vi "Velocity  실습.vi"() -> ()   [LabVIEW 2014]
uses:
  <vilib>/Motion/FlexMotion/CustomControls/CustomControls.llb/AxisOrVectorSpace To Configure.flx
  <vilib>/Motion/FlexMotion/FunctionsVIs/Trajectory.llb/Load Acceleration/Deceleration.flx
  <vilib>/Motion/FlexMotion/FunctionsVIs/StartStopMotion.llb/Start Motion (8 axes).flx
  <vilib>/Motion/FlexMotion/FunctionsVIs/StartStopMotion.llb/Stop Motion (8 axes).flx
panel:
  in  "정지":bool
  in  "Velocity (10000)":i32=3600 min=-20000000 max=20000000
  in  "Acceleration (100000)":u32=36000
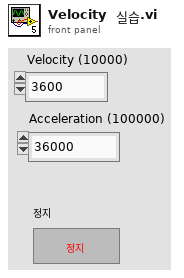
[diagram p1: front panel]
types:
  T1 = enum16{"Absolute Position", "Relative Position", "Velocity", "Relative to Cap Pos", "Modulus Position", "Absolute Contouring", "Relative Contouring"}
  T2 = typedef "AxisOrVectorSpace To Configure.flx" = u16
  T3 = typedef "Resource Out (Enum).flx" = u16
  T4 = typedef "Bd Id Out" = u8
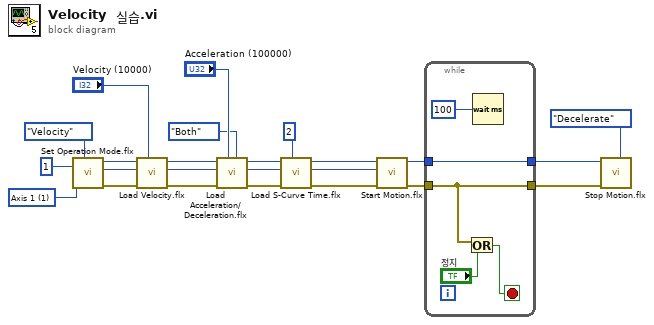
[diagram p0: block diagram]
diagram:
  w24 = T2 1 items=["Axis 1"=1, "Axis 2"=2, "Axis 3"=3, "Axis 4"=4, "Axis 5"=5, "Axis 6"=6, "Axis 7"=7, "Axis 8"=8, "Vector Space 1"=17, "Vector Space 2"=18, "Vector Space 3"=19, "Vector Space 4"=20] ("Axis or Vector Space")
  n1 = call <vilib>:"Set Operation Mode.flx"("Position Mode (Absolute)"=T1."Velocity", "Axis or Vector Space"=w24, "Board ID"=u8 1) -> ("error out"=w12:errorcluster, "Resource Output"=w13:T3, "Bd ID Out"=w14:T4)  [unwired: 3 in]
  n2 = call <vilib>:"Load Velocity.flx"("Velocity (10000)"="Velocity (10000)", "error in (no error)"=w12, "Axis or Vector Space"=w13, "Board ID"=w14) -> ("error out"=w8:errorcluster, "Resource Output"=w9:T3, "Bd ID Out"=w10:T4)  [unwired: 3 in]
  n3 = call "Load Acceleration/Deceleration.flx"("Acceleration Type (Both)"=enum16{"Both", "Acceleration", "Deceleration"}."Both", "Acceleration (100000)"="Acceleration (100000)", "error in (no error)"=w8, "Axis or Vector Space"=w9, "Board ID"=w10) -> ("error out"=w18:errorcluster, "Resource Output"=w19:T3, "Bd ID Out"=w20:T4)  [unwired: 2 in]
  n4 = call <vilib>:"Load S-Curve Time.flx"("S Curve Time (1)"=u16 2, "error in (no error)"=w18, "Axis or Vector Space"=w19, "Board ID"=w20) -> ("error out"=w5:errorcluster, "Resource Output"=w6:T3, "Bd ID Out"=w17:T4)  [unwired: 3 in]
  n5 = call-poly <vilib>:"Start Motion.flx"("error in (no error)"=w5, "Axis or Vector Space"=w6, "Board ID"=w17) -> ("error out"=w2:errorcluster, "Bd ID Out"=w16:T4)  [unwired: 3 in, 1 out]
  n6 = while {
    tunnel: w16 -> [w29]
    tunnel: [w29] -> w4
    tunnel: [w26] -> w3
    tunnel: w2 -> [w26]
    stop <- w25 stop-if-true
    n7 = Or(x=w26, y="정지") -> (x .or. y?=w25:bool)
    n8 = Wait (ms)(milliseconds to wait=u32 100 ("대기 시간(ms)")) -> ()  [unwired: 1 out]
  }
  n9 = call-poly <vilib>:"Stop Motion.flx"("Stop Type (Decel)"=enum16{"Decelerate", "Halt", "Kill"}."Decelerate", "error in (no error)"=w3, "Board ID"=w4) -> ()  [unwired: 4 in, 3 out]
